vi "Stop_Signal_State.vi"(8 "error in (no error)":errorcluster, 10 "Stop Signal":bool, 11 "USB-87Pn_Data":T1) -> (0 "error out":errorcluster, 3 "USB-87Pn_Data out":T1)   [LabVIEW 2019, in "USB-87P8_Manager.lvlib"]
uses:
  Module/USB-87P8_Manager.lvlib
  USB-87Pn_Data.ctl
  USB-87Pn.lvclass
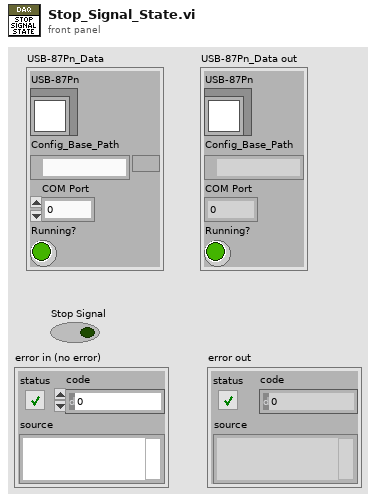
[diagram p1: front panel]
types:
  T1 = typedef "USB-87P8_Manager.lvlib/USB-87Pn_Data.ctl" = cluster{"USB-87Pn":refnum<class "USB-87Pn.lvclass">, "Config_Base_Path":path, "COM Port":i32, "Running?":bool}
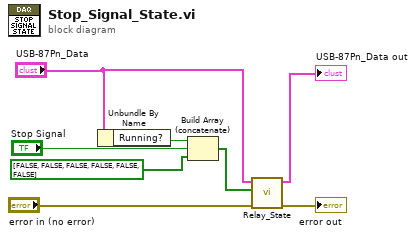
[diagram p0: block diagram]
diagram:
  n1 = Unbundle By Name("USB-87Pn_Data") -> ("Running?"=w4:bool)
  n2 = Build Array (concatenate)(w4, "Stop Signal", bool[] [FALSE, FALSE, FALSE, FALSE, FALSE, FALSE]) -> (w1:bool[])
  n3 = call "Relay_State.vi"("error in (no error)"="error in (no error)", "Relay_States"=w1, "USB-87Pn_Data In"="USB-87Pn_Data") -> ("error out"=→"error out":errorcluster, "USB-87Pn_Data Out"=→"USB-87Pn_Data out":T1)  [unwired: 7 in]
